vi "GetDryStorageContent.vi"() -> (0 "DB Serial Nos.":string[](array[string]), 1 "Channel Nos.":string[](array[string]))   [LabVIEW 2013]
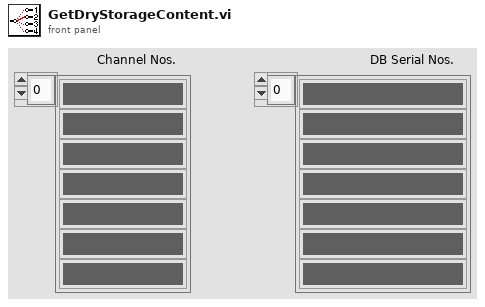
[diagram p1: front panel]
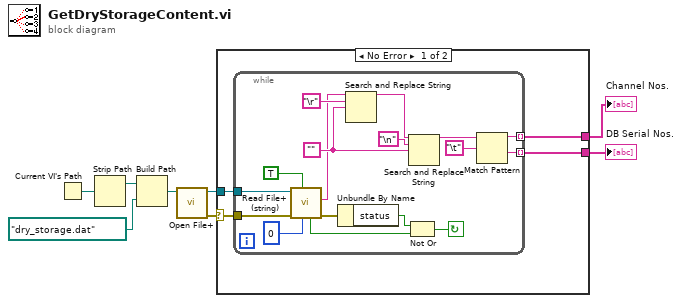
[diagram p0: block diagram]
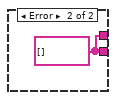
[diagram p2: hidden frame]
diagram:
  n1 = Current VI's Path() -> (path=w7:path)
  n2 = Strip Path(path=w7) -> (stripped path=w8:path)  [unwired: 1 out]
  n3 = Build Path(base path=w8, name or relative path=path "dry_storage.dat") -> (appended path=w5:path)
  n4 = call <vilib>:"Open File+.vi"("file path (\" \")"=w5) -> ("error out"=w4:errorcluster, "refnum"=w3:refnum<file>)  [unwired: 7 in, 2 out]
  n5 = case shown="No Error" w4 {
    selector: w4 -> [w11 _]
    tunnel: w3 -> [w12 _]
    tunnel: [w10 w30] -> w2
    tunnel: [w9 w30] -> w1
    frame No Error {
      n6 = while {
        tunnel: w12 -> [w29]
        tunnel: w11 -> [w28]
        tunnel: [w18] -> w10 mode=indexing
        tunnel: [w17] -> w9 mode=indexing
        stop <- w14 continue-if-true
        w25 = ""
        n7 = call <vilib>:"Read File+ (string).vi"("count"=0, "line mode (characters:F)"=TRUE, "error in (no error)"=w28, "refnum"=w29) -> ("error out"=w22:errorcluster, "string"=w21:string, "EOF?"=w15:bool)  [unwired: 3 in, 2 out]
        n8 = Unbundle By Name(w22) -> ("status"=w16:bool)
        n9 = Search and Replace String(input string=w21, search string="\r", replace string=w25) -> (result string=w24:string)  [unwired: 5 in, 3 out]
        n10 = Not Or(1:w15, 2:w16) -> (0:w14:bool)
        n11 = Search and Replace String(input string=w24, search string="\n", replace string=w25) -> (result string=w19:string)  [unwired: 5 in, 3 out]
        n12 = Match Pattern(string=w19, regular expression="\t") -> (before substring=w17:string, after substring=w18:string)  [unwired: 1 in, 2 out]
      }
    }
    frame Error {
      w30 = string[] []
    }
  }
  "Channel Nos." <- w1
  "DB Serial Nos." <- w2
